vi "ilemt_globals.vi"() -> ()   [LabVIEW 2014]
uses:
  modulation_info.ctl
panel:
  in  "TCP output connection":refnum<k5>
  in  "Ref carrier ampl":cdb[][][](array[numeric])=[[[1.0+0.0i, 1.0+0.0i, 1.0+0.0i], [1.0+0.0i, 1.0+0.0i, 1.0+0.0i]], [[1.0+0.0i, 1.0+0.0i, 1.0+0.0i], [1.0+0.0i, 1.0+0.0i, 1.0+0.0i]]] format="%#_3p"
  in  "Carrier amplitudes":cdb[][][](array[numeric]) format="%#_4g"
  in  "Modulation info":T1={"Fs full"=0.0, "Fs high"=0.0, "Fs low"=0.0, "Read size"=5000, "FFT size low"=5000, "df low"=5000.0, "High carriers"=[], "Low carriers"=[], "Hi channels at low"=[7]} {"Hi channels at low" min=0 step=1; "Low carriers" format="%#_6p"; "High carriers" format="%#_6p"}
  in  "TCP input connection":refnum<k5>
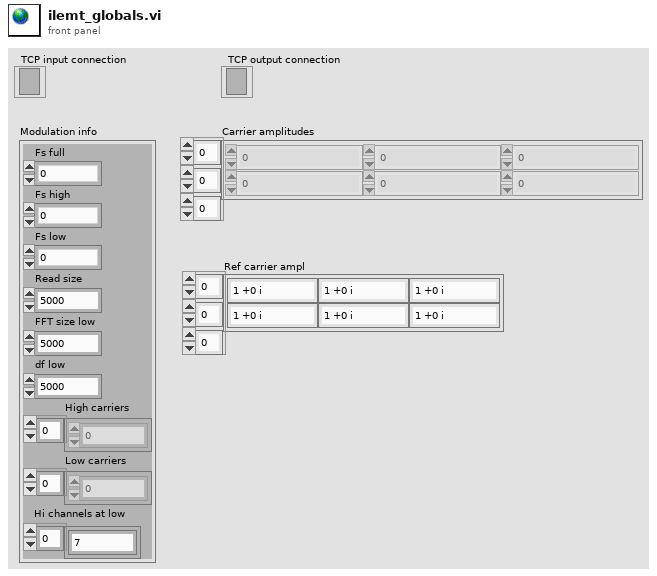
[diagram p1: front panel]
types:
  T1 = typedef "modulation_info.ctl" = cluster{"Fs full":dbl, "Fs high":dbl, "Fs low":dbl, "Read size":i32, "FFT size low":i32, "df low":dbl, "High carriers":dbl[], "Low carriers":dbl[], "Hi channels at low":i32[]}
diagram:
